vi "remove active channels speed check.vi"(9 "Data":T1={"Parameters"={"FPGA Ref"=refnum, "data stream"={"data writer name"="error writer", "NS write buffer size"=16, "NS Buffer length"=0}, "FIFO Depth"=0, "Channel controls"={"FIFIO channel count"=0, "active indices"=[], "active channels"=0, "channelScaling"=[], "scanivalveCount"=0}, "safetyChannels"={"oilP"=0, "airP"=0, "water"=0, "channelLimits"=[]}, "speedChannel"=0, "maxSpeedLimit"=0.0}, "Variables"={"Intermediary buffer"=[], "buffer position"=0, "write loop counter"=0, "NS write trigger"=0, "NS Connection status"=FALSE, "waiting for NS"=FALSE, "labAmbient"={"pressure"=0.0, "temperature"=0.0}, "scanivalvePorts"=[], "scanivalvePressures"=[], "data stream"="", "activeChannelLimitIndex"=[], "runningSpeedLimit"=0.0}}, 11 "raw data":sgl[](array[numeric])) -> (1 "data length":i32, 3 "Active channels":sgl[][](array[numeric]))   [LabVIEW 2018]
uses:
  Type Defs/channelScalingTypes.ctl
  Type Defs/scalingMethods.ctl
  Type Defs/Data processing loop data.ctl
  Type Defs/FPGA reference.ctl
  PC/type defs/channelControl.ctl
  PC/type defs/limitActions.ctl
  PC/type defs/channelLimitControl.ctl
panel:
  out "time":dbl
  out "Data received":sgl[][](array[numeric])
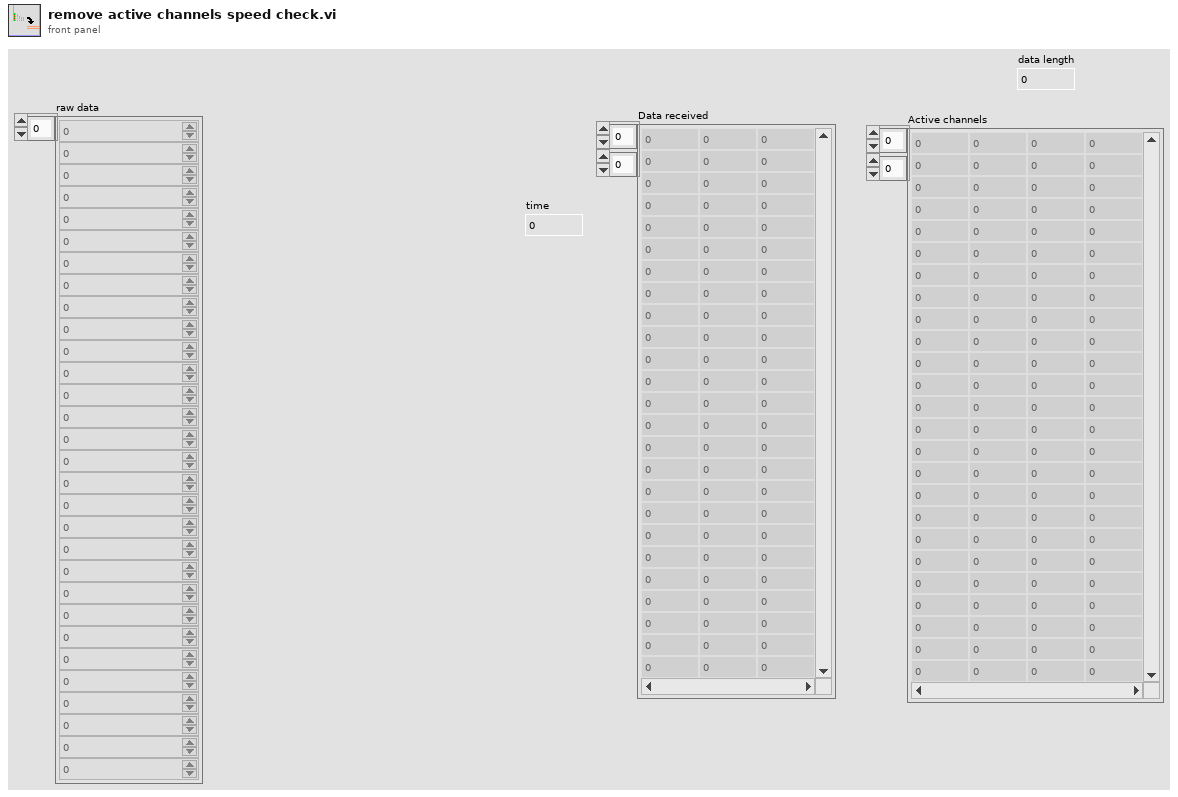
[diagram p1: front panel]
types:
  T1 = typedef "Data processing loop data.ctl" = cluster{"Parameters":cluster{"FPGA Ref":T2, "data stream":cluster{"data writer name":string, "NS write buffer size":i32, "NS Buffer length":u32}, "FIFO Depth":u32, "Channel controls":cluster{"FIFIO channel count":i32, "active indices":i16[], "active channels":i32, "channelScaling":T3[], "scanivalveCount":i32}, "safetyChannels":cluster{"oilP":u16, "airP":u16, "water":u16, "channelLimits":T6[]}, "speedChannel":i32, "maxSpeedLimit":dbl}, "Variables":cluster{"Intermediary buffer":dbl[][], "buffer position":u32, "write loop counter":u16, "NS write trigger":u32, "NS Connection status":bool, "waiting for NS":bool, "labAmbient":cluster{"pressure":dbl, "temperature":dbl}, "scanivalvePorts":u16[], "scanivalvePressures":dbl[], "data stream":refnum<k21>, "activeChannelLimitIndex":u16[], "runningSpeedLimit":dbl}}
  T2 = typedef "FPGA reference.ctl" = refnum<k20>
  T3 = typedef "channelControl.ctl" = cluster{"index":u16, "active":bool, "channelType":T4, "module":u16, "terminal":u16, "channelName":string, "scalingMethod":T5, "scalingParameters":dbl[], "scaledUnits":string, "tempOffset":dbl}
  T4 = typedef "channelScalingTypes.ctl" = enum16{"calculation", "measurement", "scanivalve", "output", "digital"}
  T5 = typedef "scalingMethods.ctl" = enum16{"none", "linear", "thermocouple", "polynomial", "encoder", "RTD"}
  T6 = typedef "channelLimitControl.ctl" = cluster{"channelID":u16, "Enabled":bool, "warnValue":dbl, "limitValue":dbl, "Invert":bool, "limitAction":T7}
  T7 = typedef "limitActions.ctl" = enum16{"stop", "shutdown", "ignore"}
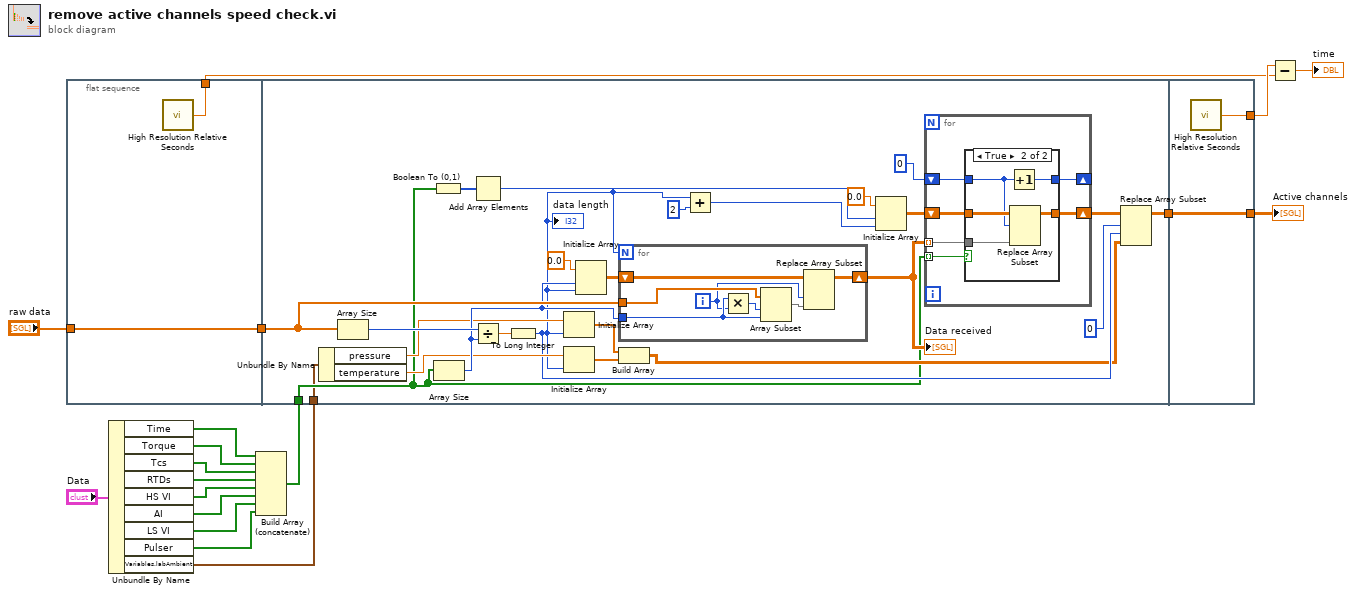
[diagram p0: block diagram]
diagram:
  n1 = flat-sequence {
    tunnel: "raw data" -> [w20]
    tunnel: [w20] -> w16
    tunnel: [w19] -> w13
    tunnel: w16 -> [w42]
    tunnel: [w28] -> w15
    tunnel: w2 -> [w22]
    tunnel: w1 -> [w21]
    tunnel: [w67] -> w17
    tunnel: w15 -> [w67]
    tunnel: [w66] -> w14
    frame #0 {
      n2 = call <vilib>:"High Resolution Relative Seconds.vi"() -> ("relative seconds"=w19:dbl)
    }
    frame #1 {
      n3 = Unbundle By Name(w21) -> ("pressure"=w32:dbl, "temperature"=w31:dbl)
      n4 = Array Size(array=w42) -> (size(s)=w45:i32)
      n5 = Boolean To (0,1)(Boolean=w22) -> (0, 1=w39:i16[])
      n6 = Array Size(array=w22) -> (size(s)=w33:i32)
      n7 = Add Array Elements(numeric array=w39) -> (sum=w37:i16)
      n8 = Divide(x=w45, y=w33) -> (x/y=w44:dbl)
      n9 = To Long Integer(number=w44) -> (32bit integer=w27:i32)
      "data length" <- w27
      n10 = Initialize Array(w32, w27) -> (w26:dbl[])
      n11 = Initialize Array(w31, w27) -> (w25:dbl[])
      n12 = Initialize Array(sgl 0.0 ("raw data"), w33, w27) -> (w41:sgl[][])
      n13 = for {
        N: w27 -> [_]
        tunnel: w42 -> [w65]
        shift-right: [w60] -> w40
        shift-left: w41 -> [w62]
        tunnel: w33 -> [w63]
        i -> [w59]
        n14 = Multiply(x=w63, y=w59) -> (x*y=w64:i32)
        n15 = Array Subset(array=w65, index=w64, length=w63) -> (w61:sgl[])
        n16 = Replace Array Subset(array=w62, new element=w61, index (col)=w59) -> (w60:sgl[][])  [unwired: 1 in]
      }
      "Data received" <- w40
      n17 = Build Array(w26, w25) -> (w24:dbl[][])
      n18 = Add(x=w27, y=2) -> (x+y=w30:i32)
      n19 = Initialize Array(sgl 0.0 ("raw data"), w37, w30) -> (w36:sgl[][])
      n20 = for {
        tunnel: w40 -> [w48] mode=indexing
        tunnel: w22 -> [w49] mode=indexing
        shift-right: [w46] -> w34
        shift-left: w36 -> [w51]
        shift-right: [w47] -> _
        shift-left: 0 ("index (row)") -> [w50]
        n21 = case shown="True" w49 {
          tunnel: w51 -> [w52 w58]
          tunnel: w50 -> [w53 w56]
          tunnel: w48 -> [_ w57]
          tunnel: [w53 w55] -> w47
          tunnel: [w52 w54] -> w46
          frame False {
          }
          frame True {
            n22 = Increment(x=w56) -> (x+1=w55:i32)
            n23 = Replace Array Subset(array=w58, new element=w57, index (row)=w56) -> (w54:sgl[][])  [unwired: 1 in]
          }
        }
      }
      n24 = Replace Array Subset(array=w34, new element=w24, index (row)=0 ("disabled index (row)"), index (col)=w27) -> (w28:sgl[][])
    }
    frame #2 {
      n25 = call <vilib>:"High Resolution Relative Seconds.vi"() -> ("relative seconds"=w66:dbl)
    }
  }
  n26 = Unbundle By Name("Data") -> ("Time"=w5:bool[], "Torque"=w4:bool[], "Tcs"=w11:bool[], "RTDs"=w10:bool[], "HS VI"=w9:bool[], "AI"=w8:bool[], "LS VI"=w7:bool[], "Pulser"=w6:bool[], "Variables.labAmbient"=w1:cluster{"pressure":dbl, "temperature":dbl})
  n27 = Build Array (concatenate)(w5, w4, w11, w10, w9, w8, w7, w6) -> (w2:bool[])
  n28 = Subtract(x=w14, y=w13) -> (x-y=→"time":dbl)
  "Active channels" <- w17
